vi "Scripting Example.vi"(7 "Server Alias":string, 10 "Ports":T1={"KA Port (9007)"=9007, "LtoP Port (9008)"=9008, "PtoL Port (9009)"=9009}, 11 "Local IP Address for LabVIEW Server":string="localhost") -> ()   [LabVIEW 2013]
doc: "This is the Scripting Example.vi, which serves as a template for the user. You have a number of Method VI's you can call (that are not in the Private section of the TS.lvlib). Notice that the Pet Server VI has to be run in its own loop, so that any GUI elements do not block that VI from running."
uses:
  LabVIEW Core/TS.lvlib
  LabVIEW Core/LabVIEW Python Connector Message.ctl
  Supporting Code/Script Running.ctl
  LabVIEW Core/Ports - Keep-Alive, LabVIEW-to-Python, Python-to-LabVIEW.ctl
panel:
  in  "Run Script":bool
  in  "Clear Status":bool
  in  "Tell Local Python the IP Address of LabVIEW Server":string="localhost"
  in  "Script ID to Abort":i64
  out "All Scripts":T2[](array[typedef])
  in  "Enable Scrolling?":bool=TRUE
  out "Unhandled Command":string
  in  "Path to python.exe (optional)":path
  in  "Abort Script":bool
  out "Script Status":string
  in  "Quit Python":bool
  in  "Launch Python":bool
  out "Connected to Python":bool
  in  "Hide Window":bool
  in  "Show Window":bool
  in  "Send":bool
  in  "LabVIEW to Python":T3={"Command"="Hello, Python!", "Data"=["Hello", "Python!"], "Script ID"=0, "LabVIEW Server ID"="localhost:9007", "Python Message ID"=0}
  out "Messages Received":i32
  out "Python to LabVIEW":T3={"Command"="", "Data"=[], "Script ID"=0, "LabVIEW Server ID"="localhost:9007", "Python Message ID"=0}
  in  "Shutdown":bool
  # "Initialize and Shutdown Python"
  # "Scripting"
  # "No Python function \n(Show Window, Hide\nWindow, Send, Run Script,\nAbort Script, Quit Python)\nwill work until after the \"Connected to Python\" LED lights up."
  # "Basic Messaging (debugging)"
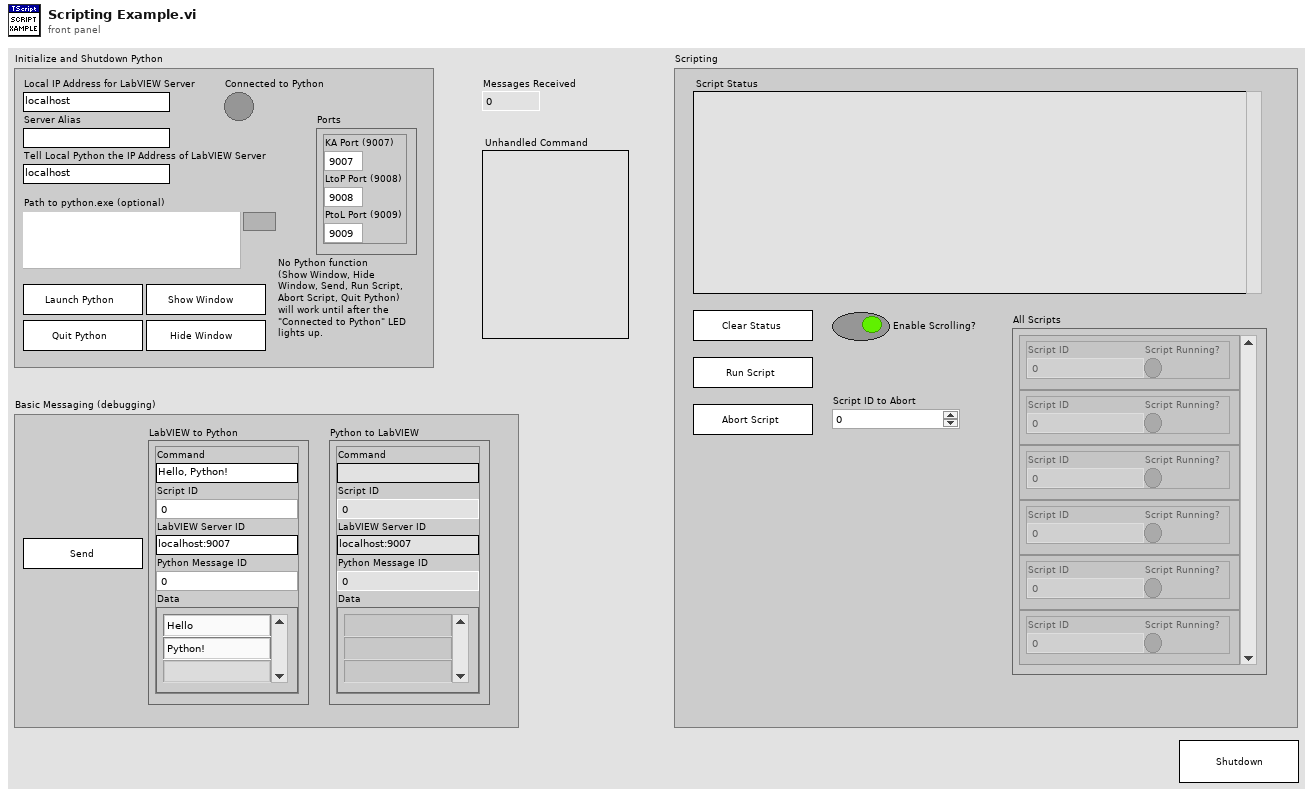
[diagram p1: front panel]
types:
  T1 = typedef "TS.lvlib/Ports - Keep-Alive, LabVIEW-to-Python, Python-to-LabVIEW.ctl" = cluster{"KA Port (9007)":u16, "LtoP Port (9008)":u16, "PtoL Port (9009)":u16}
  T2 = typedef "TS.lvlib/Script Running.ctl" = cluster{"Script ID":i64, "Script Running?":bool}
  T3 = typedef "TS.lvlib/LabVIEW Python Connector Message.ctl" = cluster{"Command":string, "Data":string[], "Script ID":i64, "LabVIEW Server ID":string, "Python Message ID":i32}
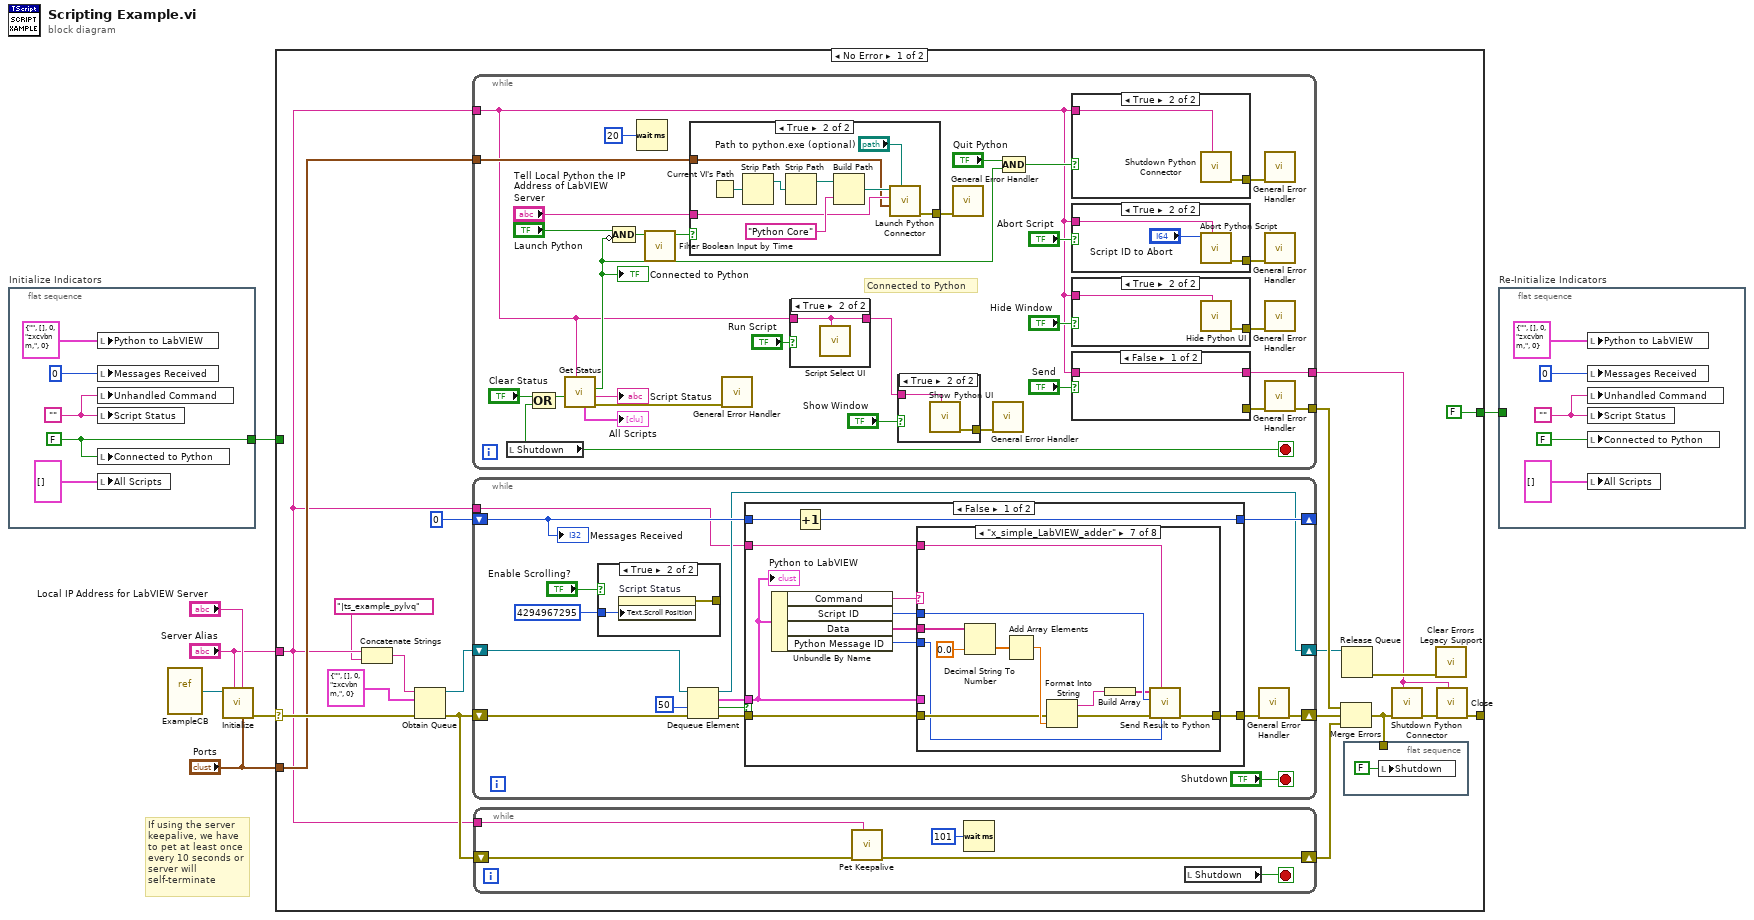
[diagram p0: block diagram]
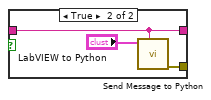
[diagram p8: hidden frame]
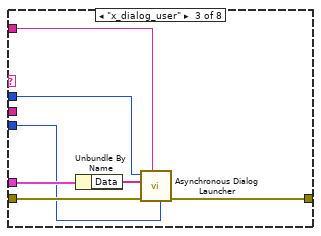
[diagram p12: hidden frame]
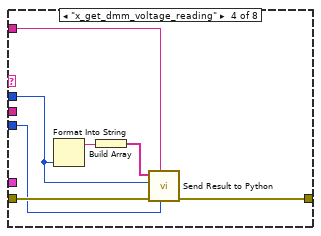
[diagram p13: hidden frame]
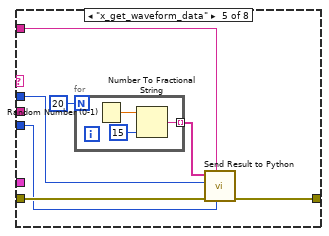
[diagram p14: hidden frame]
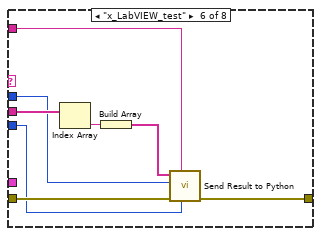
[diagram p15: hidden frame]
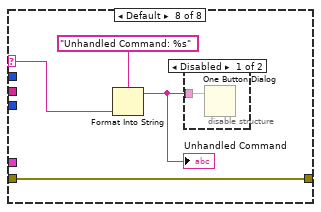
[diagram p16: hidden frame]
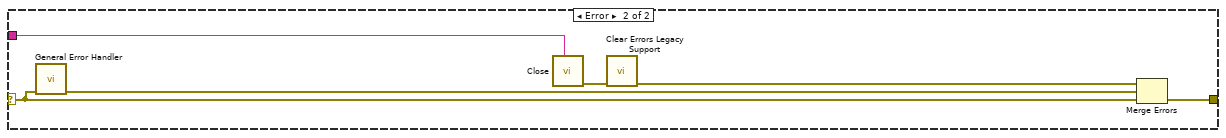
[diagram p19: hidden frame]
diagram:
  # "If using the server\nkeepalive, we have\nto pet at least once\nevery 10 seconds or\nserver will \nself-terminate"
  n1 = flat-sequence "Initialize Indicators" {
    tunnel: [w8] -> w5
    frame #0 {
      w11 = ""
      w8 = FALSE
      n2 = local write "Python to LabVIEW"(T3 {"Command"="", "Data"=[], "Script ID"=0, "LabVIEW Server ID"="zxcvbnm,", "Python Message ID"=0} ("Python to LabVIEW")) -> ()
      n3 = local write "Messages Received"(0 ("Messages Received")) -> ()
      n4 = local write "Unhandled Command"(w11) -> ()
      n5 = local write "Script Status"(w11) -> ()
      n6 = local write "Connected to Python"(w8) -> ()
      n7 = local write "All Scripts"(T2[] [] ("All Scripts")) -> ()
    }
  }
  n8 = vi-ref "ExampleCB.vi"() -> (w1:refnum<vi>)
  n9 = call "Initialize.vi"("Ports"="Ports", "IP Address for LabVIEW Server"="Local IP Address for LabVIEW Server", "Server Alias"="Server Alias", "VI Refnum"=w1) -> ("error out"=w3:errorcluster)  [unwired: 7 in]
  n10 = case shown="No Error" w3 {
    selector: w3 -> [w24 w176]
    tunnel: [FALSE _] -> w6
    tunnel: w5 -> [_ _]
    tunnel: "Ports" -> [w21 _]
    tunnel: [w20 w173] -> _
    tunnel: "Server Alias" -> [w15 w172]
    frame No Error {
      n11 = Concatenate Strings(w15, "|ts_example_pylvq" ("name (unnamed)")) -> (w13:string)
      n12 = Obtain Queue(name (unnamed)=w13, element data type=T3 {"Command"="", "Data"=[], "Script ID"=0, "LabVIEW Server ID"="zxcvbnm,", "Python Message ID"=0} ("element"), error in (no error)=w24) -> (queue out=w19:refnum<queue>, error out=w27:errorcluster)  [unwired: 2 in, 1 out]
      n13 = while {
        tunnel: [w39] -> w23
        tunnel: w21 -> [w36]
        tunnel: w15 -> [w34]
        tunnel: [w35] -> w16
        stop <- w37 stop-if-true
        # "Connected to Python"
        n14 = local read "Shutdown"() -> (w37:bool)
        n15 = Compound Arithmetic op=OR("Clear Status", w37) -> (w38:bool)
        n16 = call "Get Status.vi"("Server Alias"=w34, "Clear Status? (F)"=w38) -> ("error out"=w55:errorcluster, "Script Status"=→"Script Status":string, "Connected"=w57:bool, "All Scripts"=→"All Scripts":T2[])  [unwired: 4 in, 2 out]
        "Connected to Python" <- w57
        n17 = Compound Arithmetic op=AND("Launch Python", invert w57) -> (w60:bool)
        n18 = Wait (ms)(milliseconds to wait=u32 20) -> ()  [unwired: 1 out]
        n19 = call "Filter Boolean Input by Time.vi"("Boolean In"=w60) -> ("Boolean Out"=w61:bool)  [unwired: 10 in]
        n20 = case shown="True" w61 {
          tunnel: [_ w71] -> w49
          tunnel: "Tell Local Python the IP Address of LabVIEW Server" -> [_ w70]
          tunnel: w36 -> [_ w69]
          frame False {
            # "Python can be launched\nfrom outside; we don't \nwant the user to launch\nPython again if we are\nconnected from outside\nLabVIEW."
          }
          frame True {
            n21 = Current VI's Path() -> (path=w77:path)
            n22 = Strip Path(path=w77) -> (stripped path=w74:path)  [unwired: 1 out]
            n23 = Strip Path(path=w74) -> (stripped path=w73:path)  [unwired: 1 out]
            n24 = Build Path(base path=w73, name or relative path="Python Core") -> (appended path=w75:path)
            n25 = call "Launch Python Connector.vi"("Path to python.exe"="Path to python.exe (optional)", "Ports"=w69, "Tell Python the IP Address Where LabVIEW Is"=w70, "Path to Python Core Folder"=w75) -> ("error out"=w71:errorcluster)  [unwired: 7 in]
          }
        }
        n26 = call <vilib>:"General Error Handler.vi"("error in (no error)"=w55) -> ()  [unwired: 10 in, 5 out]
        n27 = case shown="True" "Run Script" {
          tunnel: w34 -> [w62 w63]
          tunnel: [w62 w63] -> w33
          frame False {
          }
          frame True {
            n28 = call "Script Select UI.vi"("Server Alias"=w63) -> ()  [unwired: 11 in]
          }
        }
        n29 = case shown="True" "Show Window" {
          tunnel: [_ w81] -> w54
          tunnel: w33 -> [_ w80]
          frame False {
          }
          frame True {
            n30 = call "Show Python UI.vi"("Server Alias"=w80) -> ("error out"=w81:errorcluster)  [unwired: 10 in]
          }
        }
        n31 = call <vilib>:"General Error Handler.vi"("error in (no error)"=w49) -> ()  [unwired: 10 in, 5 out]
        n32 = call <vilib>:"General Error Handler.vi"("error in (no error)"=w54) -> ()  [unwired: 10 in, 5 out]
        n33 = Compound Arithmetic op=AND("Quit Python", w57) -> (w59:bool)
        n34 = case shown="True" w59 {
          tunnel: [_ w68] -> w53
          tunnel: w34 -> [_ w67]
          frame False {
            # "Python can be quit from outside; if so, we don't \nwant the LV user to queue up another quit"
          }
          frame True {
            n35 = call "Shutdown Python Connector.vi"("Server Alias"=w67) -> ("error out"=w68:errorcluster)  [unwired: 10 in]
          }
        }
        n36 = case shown="True" "Abort Script" {
          tunnel: [_ w65] -> w52
          tunnel: w34 -> [_ w64]
          frame False {
          }
          frame True {
            n37 = call "Abort Python Script.vi"("Server Alias"=w64, "Script ID to Abort"="Script ID to Abort") -> ("error out"=w65:errorcluster)  [unwired: 9 in]
          }
        }
        n38 = case shown="True" "Hide Window" {
          tunnel: [_ w79] -> w51
          tunnel: w34 -> [_ w78]
          frame False {
          }
          frame True {
            n39 = call "Hide Python UI.vi"("Server Alias"=w78) -> ("error out"=w79:errorcluster)  [unwired: 10 in]
          }
        }
        n40 = case shown="False" "Send" {
          tunnel: [_ w84] -> w50
          tunnel: w34 -> [w82 w83]
          tunnel: [w82 w83] -> w35
          frame False {
          }
          frame True {
            n41 = call "Send Message to Python.vi"("Server Alias"=w83, "Message"="LabVIEW to Python") -> ("error out"=w84:errorcluster)  [unwired: 9 in]
          }
        }
        n42 = call <vilib>:"General Error Handler.vi"("error in (no error)"=w53) -> ()  [unwired: 10 in, 5 out]
        n43 = call <vilib>:"General Error Handler.vi"("error in (no error)"=w52) -> ()  [unwired: 10 in, 5 out]
        n44 = call <vilib>:"General Error Handler.vi"("error in (no error)"=w51) -> ()  [unwired: 10 in, 5 out]
        n45 = call <vilib>:"General Error Handler.vi"("error in (no error)"=w50) -> ("error out"=w39:errorcluster)  [unwired: 10 in, 4 out]
      }
      n46 = while {
        shift-right: [w95] -> w29
        shift-left: w27 -> [w105]
        shift-right: [w98] -> _
        shift-left: 0 -> [w99]
        shift-right: [w93] -> w18
        shift-left: w19 -> [w104]
        tunnel: w15 -> [w92]
        stop <- "Shutdown" stop-if-true
        n47 = case shown="True" "Enable Scrolling?" {
          tunnel: u32 4294967295 ("Text.Scroll Position") -> [_ w108]
          tunnel: [_ w107] -> _
          frame False {
          }
          frame True {
            n48 = property on="Script Status" class="Str"("Text.Scroll Position"=w108) -> (error out=w107:errorcluster)  [unwired: 2 in, 1 out]
          }
        }
        n49 = Dequeue Element(queue=w104, timeout in ms (-1)=50, error in (no error)=w105) -> (queue out=w93:refnum<queue>, element=w100:T3, timed out?=w102:bool, error out=w101:errorcluster)
        n50 = case shown="False" w102 {
          tunnel: w101 -> [w116 w171]
          tunnel: [w115 w171] -> w96
          tunnel: w100 -> [w114 _]
          tunnel: w99 -> [w118 w170]
          tunnel: [w117 w170] -> w98
          tunnel: w92 -> [w109 _]
          frame False {
            n51 = Unbundle By Name(w114) -> ("Command"=w113:string, "Script ID"=w112:i64, "Data"=w111:string[], "Python Message ID"=w110:i32)
            n52 = Increment(x=w118) -> (x+1=w117:i32)
            n53 = case shown="\"x_simple_LabVIEW_adder\"" w113 {
              selector: w113 -> [_ _ _ _ _ _ _ w165]
              tunnel: w116 -> [w119 w120 w126 w134 w139 w147 w158 w168]
              tunnel: [w119 w120 w125 w133 w138 w152 w164 w168] -> w115
              tunnel: w114 -> [_ _ w127 _ _ _ _ _]
              tunnel: w112 -> [_ _ w123 w130 w140 w148 w163 _]
              tunnel: w111 -> [_ _ _ _ _ w149 w162 _]
              tunnel: w110 -> [_ _ w122 w129 w136 w146 w154 _]
              tunnel: w109 -> [_ _ w121 w128 w135 w145 w153 _]
              frame "python_quit" {
                # "Not an unhandled command."
              }
              frame "register" {
                # "Registering happens elsewhere:\nthis is just to avoid\nnuisance messages when starting\na new script."
              }
              frame "x_dialog_user" {
                n54 = Unbundle By Name(w127) -> ("Data"=w124:string[])
                n55 = call "Asynchronous Dialog Launcher.vi"("Python Message ID"=w122, "Server Alias"=w121, "error in (no error)"=w126, "Data"=w124, "Script ID"=w123) -> ("error out"=w125:errorcluster)  [unwired: 6 in]
              }
              frame "x_get_dmm_voltage_reading" {
                n56 = Format Into String(w130) -> (resulting string=w131:string)  [unwired: 3 in, 1 out]
                n57 = Build Array(w131) -> (w132:string[])
                n58 = call "Send Result to Python.vi"("Python Message ID"=w129, "Server Alias"=w128, "error in (no error)"=w134, "Script ID"=w130, "Result Data"=w132) -> ("error out"=w133:errorcluster)  [unwired: 6 in]
              }
              frame "x_get_waveform_data" {
                n59 = for {
                  N: 20 -> [_]
                  tunnel: [w143] -> w137 mode=indexing
                  n60 = Random Number (0-1)() -> (number: 0 to 1=w144:dbl)
                  n61 = Number To Fractional String(number=w144, precision (6)=i16 15) -> (F-format string=w143:string)  [unwired: 2 in]
                }
                n62 = call "Send Result to Python.vi"("Python Message ID"=w136, "Server Alias"=w135, "error in (no error)"=w139, "Script ID"=w140, "Result Data"=w137) -> ("error out"=w138:errorcluster)  [unwired: 6 in]
              }
              frame "x_LabVIEW_test" {
                n63 = Index Array(array=w149) -> (element=w150:string)  [unwired: 1 in]
                n64 = Build Array(w150) -> (w151:string[])
                n65 = call "Send Result to Python.vi"("Python Message ID"=w146, "Server Alias"=w145, "error in (no error)"=w147, "Script ID"=w148, "Result Data"=w151) -> ("error out"=w152:errorcluster)  [unwired: 6 in]
              }
              frame "x_simple_LabVIEW_adder" {
                n66 = Decimal String To Number(string=w162, default (0L)=0.0) -> (number=w160:dbl[])  [unwired: 1 in, 1 out]
                n67 = Add Array Elements(numeric array=w160) -> (sum=w159:dbl)
                n68 = Format Into String(error in=w158, w159) -> (resulting string=w156:string, error out=w157:errorcluster)  [unwired: 2 in]
                n69 = Build Array(w156) -> (w155:string[])
                n70 = call "Send Result to Python.vi"("Python Message ID"=w154, "Server Alias"=w153, "error in (no error)"=w157, "Script ID"=w163, "Result Data"=w155) -> ("error out"=w164:errorcluster)  [unwired: 6 in]
              }
              frame Default {
                n71 = Format Into String(format string="Unhandled Command: %s", w165) -> (resulting string=w167:string)  [unwired: 2 in, 1 out]
                "Unhandled Command" <- w167
                n72 = disable-structure shown="Disabled" {
                  disable-tunnel: w167 -> [w169 _]
                  frame Disabled {
                    n73 = One Button Dialog(message=w169) -> ()  [unwired: 1 in, 1 out]
                  }
                  frame Enabled {
                  }
                }
              }
            }
            "Python to LabVIEW" <- w114
          }
          frame True {
          }
        }
        n74 = call <vilib>:"General Error Handler.vi"("error in (no error)"=w96) -> ("error out"=w95:errorcluster)  [unwired: 10 in, 4 out]
        "Messages Received" <- w99
      }
      n75 = while {
        shift-right: [w89] -> w26
        shift-left: w27 -> [w90]
        tunnel: w15 -> [w87]
        stop <- w91 stop-if-true
        n76 = call "Pet Keepalive.vi"("Server Alias"=w87, "error in (no error)"=w90) -> ("error out"=w89:errorcluster)  [unwired: 9 in]
        n77 = Wait (ms)(milliseconds to wait=u32 101) -> ()  [unwired: 1 out]
        n78 = local read "Shutdown"() -> (w91:bool)
      }
      n79 = Merge Errors(w23, w29, w26) -> (w25:errorcluster)
      n80 = Release Queue(queue=w18) -> (error out=w17:errorcluster)  [unwired: 2 in, 2 out]
      n81 = flat-sequence {
        tunnel: w25 -> [_]
        frame #0 {
          n82 = local write "Shutdown"(FALSE) -> ()
        }
      }
      n83 = call "Shutdown Python Connector.vi"("Server Alias"=w16, "error in (no error)"=w25) -> ("error out"=w28:errorcluster)  [unwired: 9 in]
      n84 = call "Clear Errors Legacy Support.vi"("error in (no error)"=w17) -> ()  [unwired: 5 in, 2 out]
      n85 = call "Close.vi"("Server Alias"=w16, "error in (no error)"=w28) -> ("error out"=w20:errorcluster)  [unwired: 9 in]
    }
    frame Error {
      n86 = call <vilib>:"General Error Handler.vi"("error in (no error)"=w176) -> ("error out"=w175:errorcluster)  [unwired: 10 in, 4 out]
      n87 = call "Close.vi"("Server Alias"=w172) -> ("error out"=w177:errorcluster)  [unwired: 10 in]
      n88 = call "Clear Errors Legacy Support.vi"("error in (no error)"=w177) -> ("error out"=w174:errorcluster)  [unwired: 5 in, 1 out]
      n89 = Merge Errors(w174, w175, w176) -> (w173:errorcluster)
    }
  }
  n90 = flat-sequence "Re-Initialize Indicators" {
    tunnel: w6 -> [_]
    frame #0 {
      w180 = ""
      n91 = local write "Python to LabVIEW"(T3 {"Command"="", "Data"=[], "Script ID"=0, "LabVIEW Server ID"="zxcvbnm,", "Python Message ID"=0} ("Python to LabVIEW")) -> ()
      n92 = local write "Messages Received"(0 ("Messages Received")) -> ()
      n93 = local write "Unhandled Command"(w180) -> ()
      n94 = local write "Script Status"(w180) -> ()
      n95 = local write "Connected to Python"(FALSE) -> ()
      n96 = local write "All Scripts"(T2[] [] ("All Scripts")) -> ()
    }
  }
